vi "TestModule.vi"(8 "error in (no error)":errorcluster) -> (0 "error out":errorcluster)   [LabVIEW 2025, in "DAQ_Module.lvlib"]
uses:
  DAQ_Module/DAQ_Module/DAQ_Module.lvlib
  Msg.ctl
  DAQ_Module/DAQ_Module/DAQ_Module/DAQ_Module.lvclass
  Module/Module/Module Messages/CoreComm Msg/CoreComm Msg.lvclass/CoreComm Msg.ctl
  <vilib>/ActorFramework/Message Enqueuer/Message Enqueuer.lvclass/Message Enqueuer.ctl
  9ae72363-4c45-4ff6-8a50-836a1603dbba.vi
  <vilib>/ActorFramework/Message Enqueuer/Enqueue.vi
  Module/Module/Module Messages/CoreComm Msg/CoreComm Msg.lvclass
  <vilib>/ActorFramework/Message Priority Queue/Priority Enqueue.vi
  <vilib>/ActorFramework/Actor/Actor.lvclass
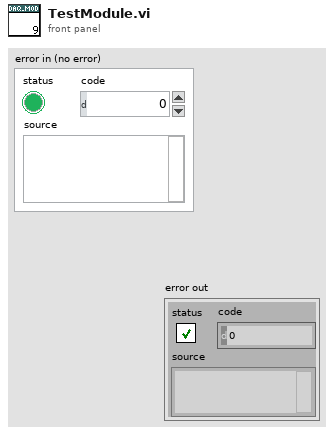
[diagram p1: front panel]
types:
  T1 = typedef "Msg.ctl" = string
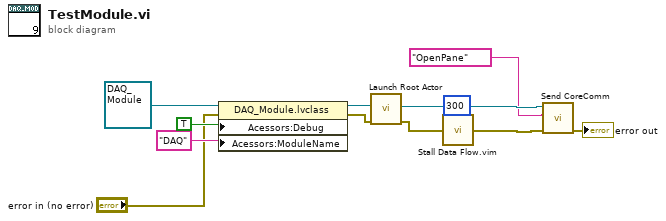
[diagram p0: block diagram]
diagram:
  n1 = property class="DAQ_Module.lvclass"(reference=refnum<class "DAQ_Module.lvclass"> refnum ("DAQ_Module.lvlib:DAQ_Module.lvclass"), error in="error in (no error)", "Acessors:Debug"=TRUE ("Debug"), "Acessors:ModuleName"="DAQ" ("ModuleName")) -> (reference out=w12:refnum<class "DAQ_Module.lvclass">, error out=w3:errorcluster)
  n2 = call <vilib>:"Launch Root Actor.vi"("error in (no error)"=w3, "Actor"=w12) -> ("error out"=w10:errorcluster, "Actor's Enqueuer"=w6:refnum<class "Message Enqueuer.lvclass">)  [unwired: 8 in]
  n3 = call "Stall Data Flow.vim"("value in"=w10, "milliseconds to wait"=u32 300) -> ("value out"=w5:errorcluster)  [unwired: 1 out]
  n4 = call "Send CoreComm.vi"("error in (no error)"=w5, "Msg"=T1 "OpenPane", "Message Enqueuer"=w6) -> ("error out"=→"error out":errorcluster)  [unwired: 7 in, 1 out]
